vi "Get_Configuration_Keithley.vi"(8 "error in":errorcluster, 11 "Filename (.ini)":string="Config_Ver_1\\Keithley_params.ini") -> (0 "error out":errorcluster, 1 "List Sweep Params In":T2={"Abort On\nCompliance?"=FALSE, "List Sweep Steps"=[{"Current Level (A)"=0.0, "Source Delay (s)"=0.001, "Voltage Limit (V)"=100.0}, {"Current Level (A)"=0.1, "Source Delay (s)"=1.0, "Voltage Limit (V)"=100.0}]} {"List Sweep Steps"."Current Level (A)" min=-0.105 max=0.105 format="%.4p"; "List Sweep Steps"."Source Delay (s)" min=0.001 max=1000.0 step=0.001 format="%.3f"; "List Sweep Steps"."Voltage Limit (V)" min=0.1 max=105.0 step=0.01 format="%.2p"}, 2 "Trig Layer Params In":T8={"Input Trig Source"=enum."Trigger Link", "Input Trig Link Line"=enum."1", "Output Trig Mode"=enum."Source Turn On", "Output Trig Link Line"=enum."2"}, 3 "Arm Layer Params In":T12={"Bypass Arm Layer\nInput Trigger?"=FALSE, "Input Trig Source"=enum."Trigger Link", "Input Trig Link Line"=enum."1", "Arm Timer Interval (s)"=0.001, "Output Trig Mode"=enum."No Trig Out", "Output Trig Link Line"=enum."1"} {"Arm Timer Interval (s)" min=0.001 max=99999.999 step=0.001 format="%.3f"}, 5 "Display Params":T1)   [LabVIEW 2021]
uses:
  <instrlib>/Keithley 622x LV 2009/Configure/Trigger/Typedefs/KE622x -- Arm Layer Params.ctl
  <instrlib>/Keithley 622x LV 2009/Configure/Trigger/Low Level/Typedefs/KE622x -- Arm Source.ctl
  <instrlib>/Keithley 622x LV 2009/Configure/Trigger/Low Level/Typedefs/KE622x -- Trig Link Line.ctl
  <instrlib>/Keithley 622x LV 2009/Configure/Trigger/Low Level/Typedefs/KE622x -- Arm Timer Interval.ctl
  <instrlib>/Keithley 622x LV 2009/Configure/Trigger/Low Level/Typedefs/KE622x -- Arm Output Mode.ctl
  <instrlib>/Keithley 622x LV 2009/Configure/Trigger/Typedefs/KE622x -- Trig Layer Params.ctl
  <instrlib>/Keithley 622x LV 2009/Configure/Trigger/Low Level/Typedefs/KE622x -- Trig Source.ctl
  <instrlib>/Keithley 622x LV 2009/Configure/Trigger/Low Level/Typedefs/KE622x -- Trig Output Mode.ctl
  <instrlib>/Keithley 622x LV 2009/Configure/Source/Typedefs/KE622x -- List Sweep Params.ctl
  <instrlib>/Keithley 622x LV 2009/Configure/Source/Typedefs/KE622x -- List Sweep Steps.ctl
  <instrlib>/Keithley 622x LV 2009/Configure/Source/Typedefs/KE622x -- List Sweep Step.ctl
  <instrlib>/Keithley 622x LV 2009/Configure/Source/Typedefs/KE622x -- Current Level.ctl
  <instrlib>/Keithley 622x LV 2009/Configure/Source/Typedefs/KE622x -- Source Delay.ctl
  <instrlib>/Keithley 622x LV 2009/Configure/Source/Typedefs/KE622x -- Voltage Limit.ctl
  <instrlib>/Keithley 622x LV 2009/Configure/Display/Typedefs/KE622x -- Display Params.ctl
  <vilib>/Utility/config.llb/NI_LVConfig.lvlib
  <instrlib>/Keithley 622x LV 2009/Keithley 622x.lvlib
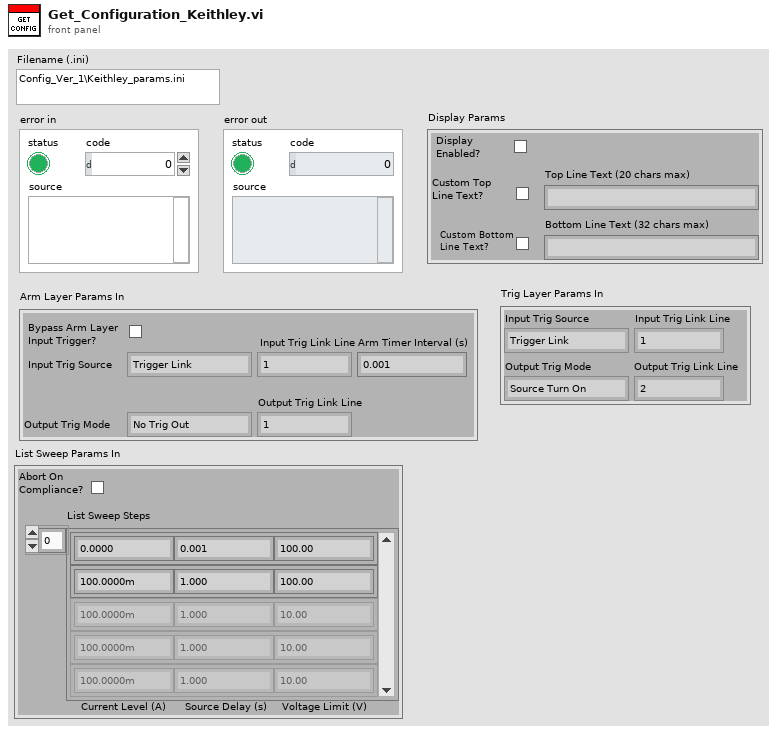
[diagram p1: front panel]
types:
  T1 = typedef "Keithley 622x.lvlib/KE622x -- Display Params.ctl" = cluster{"Display\nEnabled?":bool, "Custom Top\nLine Text?":bool, "Top Line Text (20 chars max)":string, "Custom Bottom\nLine Text?":bool, "Bottom Line Text (32 chars max)":string}
  T2 = typedef "Keithley 622x.lvlib/KE622x -- List Sweep Params.ctl" = cluster{"Abort On\nCompliance?":bool, "List Sweep Steps":T3}
  T3 = typedef "Keithley 622x.lvlib/KE622x -- List Sweep Steps.ctl" = T4[]
  T4 = typedef "Keithley 622x.lvlib/KE622x -- List Sweep Step.ctl" = cluster{"Current Level (A)":T5, "Source Delay (s)":T6, "Voltage Limit (V)":T7}
  T5 = typedef "Keithley 622x.lvlib/KE622x -- Current Level.ctl" = dbl
  T6 = typedef "Keithley 622x.lvlib/KE622x -- Source Delay.ctl" = dbl
  T7 = typedef "Keithley 622x.lvlib/KE622x -- Voltage Limit.ctl" = dbl
  T8 = typedef "Keithley 622x.lvlib/KE622x -- Trig Layer Params.ctl" = cluster{"Input Trig Source":T9, "Input Trig Link Line":T10, "Output Trig Mode":T11, "Output Trig Link Line":T10}
  T9 = typedef "Keithley 622x.lvlib/KE622x -- Trig Source.ctl" = enum16{"Immediate", "Trigger Link"}
  T10 = typedef "Keithley 622x.lvlib/KE622x -- Trig Link Line.ctl" = enum16{"1", "2", "3", "4", "5", "6"}
  T11 = typedef "Keithley 622x.lvlib/KE622x -- Trig Output Mode.ctl" = enum16{"No Trig Out", "Source Turn On", "After Source Delay"}
  T12 = typedef "Keithley 622x.lvlib/KE622x -- Arm Layer Params.ctl" = cluster{"Bypass Arm Layer\nInput Trigger?":bool, "Input Trig Source":T13, "Input Trig Link Line":T10, "Arm Timer Interval (s)":T14, "Output Trig Mode":T15, "Output Trig Link Line":T10}
  T13 = typedef "Keithley 622x.lvlib/KE622x -- Arm Source.ctl" = enum16{"Immediate", "Bus (*TRG)", "Timer", "Manual", "Trigger Link", "SOT Falling Edge", "SOT Rising Edge", "SOT Either Edge"}
  T14 = typedef "Keithley 622x.lvlib/KE622x -- Arm Timer Interval.ctl" = dbl
  T15 = typedef "Keithley 622x.lvlib/KE622x -- Arm Output Mode.ctl" = enum16{"No Trig Out", "Trig Out On Enter Arm", "Trig Out On Exit Arm"}
  T16 = typedef "NI_LVConfig.lvlib/Config Data RefNum.ctl" = refnum<k1>
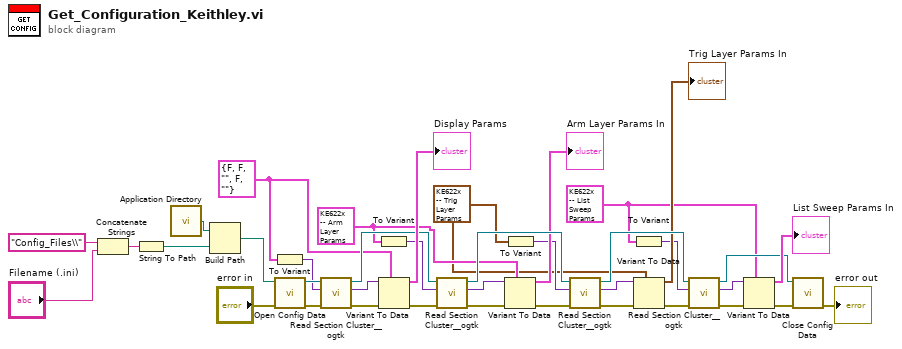
[diagram p0: block diagram]
diagram:
  w1 = T2 {"Abort On\nCompliance?"=FALSE, "List Sweep Steps"=[{"Current Level (A)"=0.0, "Source Delay (s)"=0.001, "Voltage Limit (V)"=100.0}, {"Current Level (A)"=0.1, "Source Delay (s)"=1.0, "Voltage Limit (V)"=100.0}]} ("List Sweep Params In")
  w4 = T8 {"Input Trig Source"=enum."Trigger Link", "Input Trig Link Line"=enum."1", "Output Trig Mode"=enum."Source Turn On", "Output Trig Link Line"=enum."2"} ("Trig Layer Params In")
  w7 = T12 {"Bypass Arm Layer\nInput Trigger?"=FALSE, "Input Trig Source"=enum."Trigger Link", "Input Trig Link Line"=enum."1", "Arm Timer Interval (s)"=0.001, "Output Trig Mode"=enum."No Trig Out", "Output Trig Link Line"=enum."1"} ("Arm Layer Params In")
  w10 = T1 {"Display\nEnabled?"=FALSE, "Custom Top\nLine Text?"=FALSE, "Top Line Text (20 chars max)"="", "Custom Bottom\nLine Text?"=FALSE, "Bottom Line Text (32 chars max)"=""} ("Display Params")
  n1 = Concatenate Strings("Config_Files\\" ("string"), "Filename (.ini)") -> (w38:string)
  n2 = String To Path(string=w38) -> (path=w36:path)
  n3 = call <vilib>:"Application Directory.vi"() -> ("Application Directory"=w34:path)
  n4 = Build Path(base path=w34, name or relative path=w36) -> (appended path=w35:path)
  n5 = To Variant(anything=w10) -> (Variant=w11:variant)
  n6 = call <vilib>:"Open Config Data.vi"("error in (no error)"="error in", "configuration file path"=w35) -> ("error out"=w33:errorcluster, "refnum"=w32:T16)  [unwired: 7 in, 1 out]
  n7 = call <userlib>:"Read Section Cluster__ogtk.vi"("error in (no error)"=w33, "Section Formatted Cluster Type"=w11, "refnum"=w32) -> ("error out"=w30:errorcluster, "Section Formatted Cluster"=w31:variant, "dup refnum"=w19:T16)  [unwired: 4 in, 2 out]
  n8 = To Variant(anything=w7) -> (Variant=w9:variant)
  n9 = Variant To Data(error in=w30, type=w10, Variant=w31) -> (data=→"Display Params":T1, error out=w8:errorcluster)
  n10 = call <userlib>:"Read Section Cluster__ogtk.vi"("error in (no error)"=w8, "Section Formatted Cluster Type"=w9, "refnum"=w19) -> ("error out"=w25:errorcluster, "Section Formatted Cluster"=w24:variant, "dup refnum"=w18:T16)  [unwired: 4 in, 2 out]
  n11 = Variant To Data(error in=w25, type=w7, Variant=w24) -> (data=→"Arm Layer Params In":T12, error out=w5:errorcluster)
  n12 = To Variant(anything=w4) -> (Variant=w6:variant)
  n13 = call <userlib>:"Read Section Cluster__ogtk.vi"("error in (no error)"=w5, "Section Formatted Cluster Type"=w6, "refnum"=w18) -> ("error out"=w22:errorcluster, "Section Formatted Cluster"=w23:variant, "dup refnum"=w17:T16)  [unwired: 4 in, 2 out]
  n14 = To Variant(anything=w1) -> (Variant=w3:variant)
  n15 = Variant To Data(error in=w22, type=w4, Variant=w23) -> (data=→"Trig Layer Params In":T8, error out=w2:errorcluster)
  n16 = call <userlib>:"Read Section Cluster__ogtk.vi"("error in (no error)"=w2, "Section Formatted Cluster Type"=w3, "refnum"=w17) -> ("error out"=w21:errorcluster, "Section Formatted Cluster"=w20:variant, "dup refnum"=w13:T16)  [unwired: 4 in, 2 out]
  n17 = Variant To Data(error in=w21, type=w1, Variant=w20) -> (data=→"List Sweep Params In":T2, error out=w12:errorcluster)
  n18 = call <vilib>:"Close Config Data.vi"("error in (no error)"=w12, "refnum"=w13) -> ("error out"=→"error out":errorcluster)  [unwired: 8 in, 1 out]
